vi "Timer GenerateCode.vi"(0 "XRef":T17, 1 "Terms":T14, 2 "Diagram":T13, 3 "State In":T1) -> (14 "Generated Code?":T9, 15 "Reply":T12, 16 "Fatal Error Out":T11, 17 "State Out":T1)   [LabVIEW 2021, in "myRIO Create Timer IRQ.xnode"]
uses:
  <vilib>/myRIO/Instrument Drivers/IRQ/Timer IRQ/vis/myRIO Create Timer IRQ.xnode
  <vilib>/XNodeSupport/XNodeXNodeRef.ctl
  <vilib>/XNodeSupport/XNodeTermIDPairs.ctl
  <vilib>/XNodeSupport/XNodeTermIDPair.ctl
  <vilib>/XNodeSupport/XNodeTermRef.ctl
  <vilib>/XNodeSupport/XNodeString.ctl
  <vilib>/XNodeSupport/XNodeTopLevelDiagramRef.ctl
  <vilib>/myRIO/Instrument Drivers/IRQ/Timer IRQ/vis/Timer State.ctl
  <vilib>/myRIO/Common/Instrument Driver Framework/Utilities/typedefs/myRIOXPeripheral.ctl
  <vilib>/XNodeSupport/XNodeTerm4Array.ctl
  <vilib>/XNodeSupport/XNodeTerm4.ctl
  <vilib>/XNodeSupport/XNodeVariant.ctl
  <vilib>/XNodeSupport/XNodeRect32.ctl
  <vilib>/XNodeSupport/XNodeInt.ctl
  <vilib>/XNodeSupport/XNodeBool.ctl
  <vilib>/XNodeSupport/XNodeTermDirection.ctl
  <vilib>/XNodeSupport/XNodeStringArray.ctl
  <vilib>/XNodeSupport/XNodeErrorCluster.ctl
  <vilib>/Utility/miscctls.llb/LVPositionTypeDef.ctl
  <vilib>/userdefined/High Color/nirio_resource_hc.ctl
  <vilib>/XNodeSupport/NI_XNodeSupport.lvlib
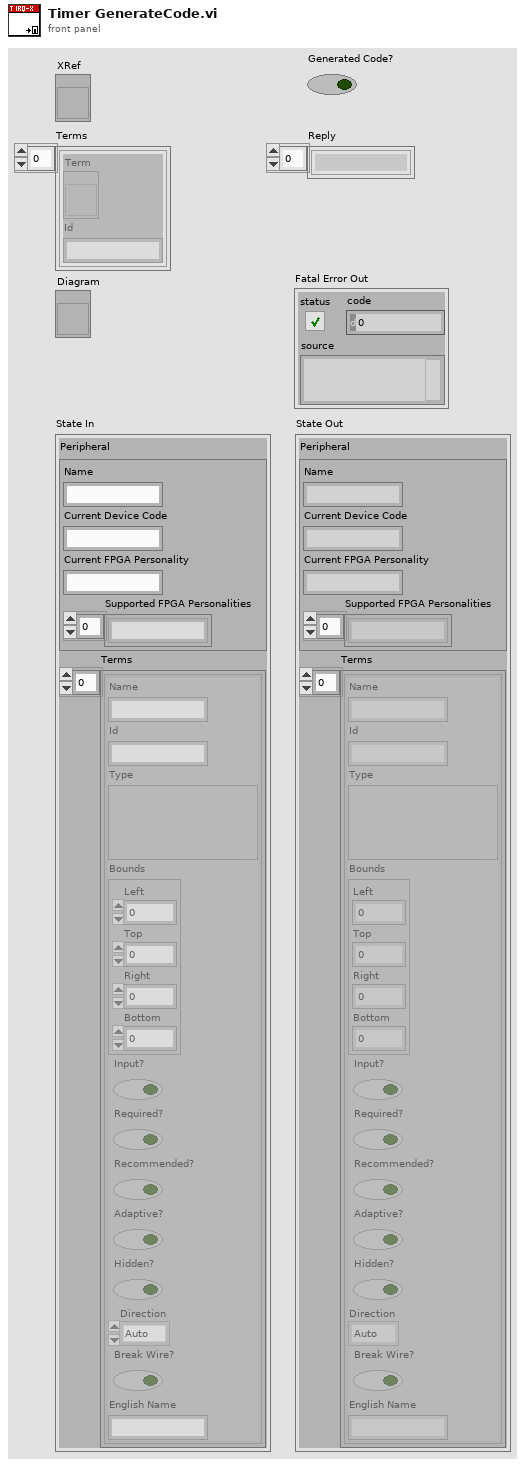
[diagram p1: front panel]
types:
  T1 = typedef "myRIO Create Timer IRQ.xnode/Timer State.ctl" = cluster{"Peripheral":T2, "Terms":T3}
  T2 = typedef "myRIOXPeripheral.ctl" = cluster{"Name":string, "Current Device Code":string, "Current FPGA Personality":string, "Supported FPGA Personalities":string[]}
  T3 = typedef "NI_XNodeSupport.lvlib/XNodeTerm4Array.ctl" = T4[]
  T4 = typedef "NI_XNodeSupport.lvlib/XNodeTerm4.ctl" = cluster{"Name":T5, "Id":T5, "Type":T6, "Bounds":T7, "Input?":T9, "Required?":T9, "Recommended?":T9, "Adaptive?":T9, "Hidden?":T9, "Direction":T10, "Break Wire?":T9, "English Name":T5}
  T5 = typedef "NI_XNodeSupport.lvlib/XNodeString.ctl" = string
  T6 = typedef "NI_XNodeSupport.lvlib/XNodeVariant.ctl" = variant
  T7 = typedef "NI_XNodeSupport.lvlib/XNodeRect32.ctl" = cluster{"Left":T8, "Top":T8, "Right":T8, "Bottom":T8}
  T8 = typedef "NI_XNodeSupport.lvlib/XNodeInt.ctl" = i32
  T9 = typedef "NI_XNodeSupport.lvlib/XNodeBool.ctl" = bool
  T10 = typedef "NI_XNodeSupport.lvlib/XNodeTermDirection.ctl" = enum32{"Auto", "Up", "Down", "Left", "Right", "Center"}
  T11 = typedef "NI_XNodeSupport.lvlib/XNodeErrorCluster.ctl" = errorcluster
  T12 = typedef "NI_XNodeSupport.lvlib/XNodeStringArray.ctl" = T5[]
  T13 = typedef "NI_XNodeSupport.lvlib/XNodeTopLevelDiagramRef.ctl" = refnum<vi>
  T14 = typedef "NI_XNodeSupport.lvlib/XNodeTermIDPairs.ctl" = T15[]
  T15 = typedef "NI_XNodeSupport.lvlib/XNodeTermIDPair.ctl" = cluster{"Term":T16, "Id":T5}
  T16 = typedef "NI_XNodeSupport.lvlib/XNodeTermRef.ctl" = refnum<vi>
  T17 = typedef "NI_XNodeSupport.lvlib/XNodeXNodeRef.ctl" = refnum<vi>
  T18 = typedef "LVPositionTypeDef.ctl" = cluster{"Left":i32, "Top":i32}
  T19 = typedef "nirio_resource_hc.ctl" = tag
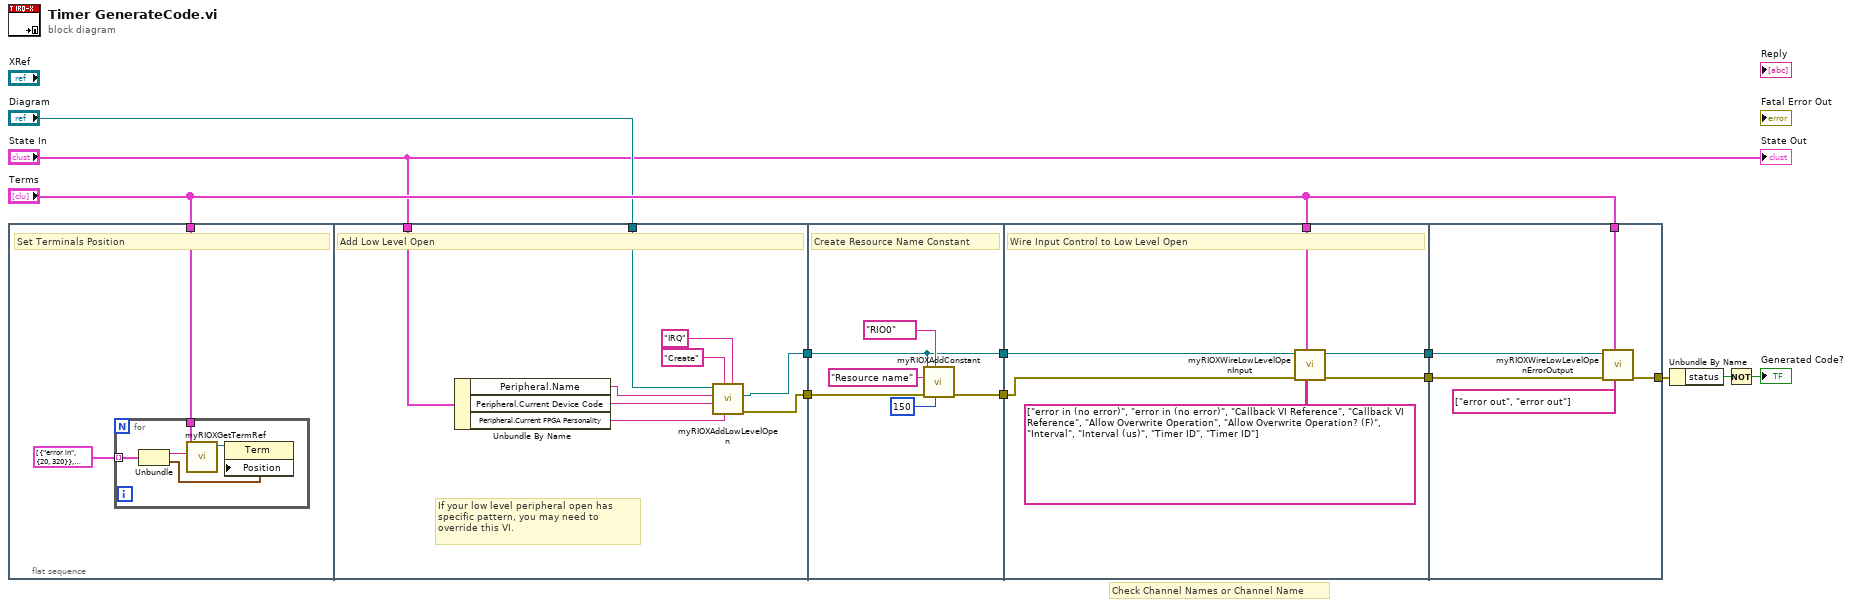
[diagram p0: block diagram]
diagram:
  # "Check Channel Names or Channel Name"
  n1 = flat-sequence {
    tunnel: "Terms" -> [w14]
    tunnel: "State In" -> [w28]
    tunnel: "Diagram" -> [w26]
    tunnel: [w24] -> w7
    tunnel: [w25] -> w6
    tunnel: [w29] -> w12
    tunnel: [w31] -> w8
    tunnel: w7 -> [w30]
    tunnel: w6 -> [w29]
    tunnel: w12 -> [w39]
    tunnel: "Terms" -> [w40]
    tunnel: [w38] -> w11
    tunnel: [w37] -> w10
    tunnel: w8 -> [w36]
    tunnel: [w44] -> w5
    tunnel: w11 -> [w45]
    tunnel: w10 -> [w43]
    tunnel: "Terms" -> [w42]
    frame #0 {
      # "Set Terminals Position"
      n2 = for {
        tunnel: w14 -> [w19]
        tunnel: cluster{"Term ID":string, "Position":T18}[] [{"Term ID"="error in", "Position"={"Left"=20, "Top"=320}}, {"Term ID"="error out", "Position"={"Left"=350, "Top"=320}}, {"Term ID"="Callback VI", "Position"={"Left"=20, "Top"=380}}, {"Term ID"="Allow Overwrite", "Position"={"Left"=20, "Top"=200}}, {"Term ID"="Interval(us)", "Position"={"Left"=20, "Top"=350}}, {"Term ID"="Timer ID", "Position"={"Left"=20, "Top"=230}}] ("Term ID Postion") -> [w17] mode=indexing
        n3 = Unbundle(w17) -> ("Term ID"=w16:string, "Position"=w15:T18)
        n4 = call <vilib>:"myRIOXGetTermRef.vi"("Term ID"=w16, "Terms"=w19) -> ("Terminal Reference"=w18:T16)  [unwired: 7 in, 2 out]
        n5 = property class="Term"(reference=w18, "Position"=w15) -> ()  [unwired: 1 in, 2 out]
      }
    }
    frame #1 {
      # "If your low level peripheral open has specific pattern, you may need to override this VI."
      # "Add Low Level Open"
      n6 = Unbundle By Name(w28) -> ("Peripheral.Name"=w21:string, "Peripheral.Current Device Code"=w23:string, "Peripheral.Current FPGA Personality"=w20:string)
      n7 = call <vilib>:"myRIOXAddLowLevelOpen.vi"("Peripheral Name"="IRQ", "FPGA Personality"=w20, "Open VI type (Open)"="Create", "Device Code"=w23, "VI Name"=w21, "Diagram Reference"=w26) -> ("error out"=w24:errorcluster, "SubVI Reference"=w25:refnum<vi>)  [unwired: 3 in, 1 out]
    }
    frame #2 {
      # "Create Resource Name Constant"
      n8 = call <vilib>:"myRIOXAddConstant.vi"("Left (0)"=150 ("Left"), "Value"=T19 "RIO0" ("Resource name"), "error in (no error)"=w30, "Terminal Name"="Resource name", "Owner Reference"=w29) -> ("error out"=w31:errorcluster)  [unwired: 5 in, 1 out]
    }
    frame #3 {
      # "Wire Input Control to Low Level Open"
      n9 = call <vilib>:"myRIOXWireLowLevelOpenInput.vi"("Wiring Specs"=string[][] [["error in (no error)", "error in (no error)"], ["Callback VI Reference", "Callback VI Reference"], ["Allow Overwrite Operation", "Allow Overwrite Operation? (F)"], ["Interval", "Interval (us)"], ["Timer ID", "Timer ID"]], "Terms"=w40, "error in (no error)"=w36, "SubVI Reference"=w39) -> ("error out"=w38:errorcluster, "Duplicated SubVI Reference"=w37:refnum<vi>)  [unwired: 6 in]
    }
    frame #4 {
      n10 = call <vilib>:"myRIOXWireLowLevelOpenErrorOutput.vi"("Wiring Specs"=string[] ["error out", "error out"], "Terms"=w42, "error in (no error)"=w45, "SubVI Reference"=w43) -> ("error out"=w44:errorcluster)  [unwired: 6 in, 1 out]
    }
  }
  n11 = Unbundle By Name(w5) -> ("status"=w1:bool)
  n12 = Not(x=w1) -> (.not. x?=→"Generated Code?":bool)
  "State Out" <- "State In"
